vi "poly_control_signalling_write_self_single.vi"(6 "mode (Sgnl)":T1(ring)=enum."Val(Sgnl)", 8 "error in (no error)":errorcluster, 9 "Value":variant, 10 "Control Name":string) -> (0 "error out":errorcluster, 2 "controll reference out":refnum<vi>, 4 "found?":bool)   [LabVIEW 2015]
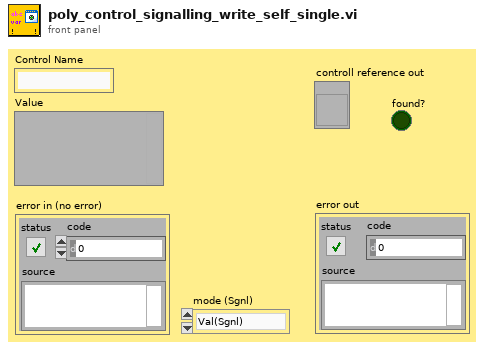
[diagram p1: front panel]
types:
  T1 = enum16{"Val", "Val(Sgnl)", "Val(Undo)", "Method"}
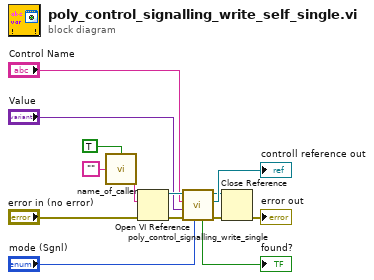
[diagram p0: block diagram]
diagram:
  n1 = call "name_of_caller.vi"("is in inlined vi? (F)"=TRUE, "name of caller in"="") -> ("name of caller out"=w13:string)  [unwired: 2 in]
  n2 = Open VI Reference(vi path=w13, error in (no error)="error in (no error)") -> (vi reference=w11:refnum<vi>, error out=w12:errorcluster)  [unwired: 4 in]
  n3 = call "poly_control_signalling_write_single.vi"("mode (Sgnl)"="mode (Sgnl)", "error in (no error)"=w12, "Value"="Value", "Control Name"="Control Name", "vi reference"=w11) -> ("error out"=w3:errorcluster, "controll reference out"=→"controll reference out":refnum<vi>, "vi reference out"=w4:refnum<vi>, "found?"=→"found?":bool)  [unwired: 3 in]
  n4 = Close Reference(reference=w4, error in (no error)=w3) -> (error out=→"error out":errorcluster)
